vi "Pockels Cal-Cal subset info from graph.vi"(8 "error in (no error)":errorcluster, 11 "XYGraph in":refnum<vi>) -> (0 "error out":errorcluster, 1 "Cal subset info array":string[][](array[string]), 3 "XYGraph":refnum<vi>)   [LabVIEW 2020]
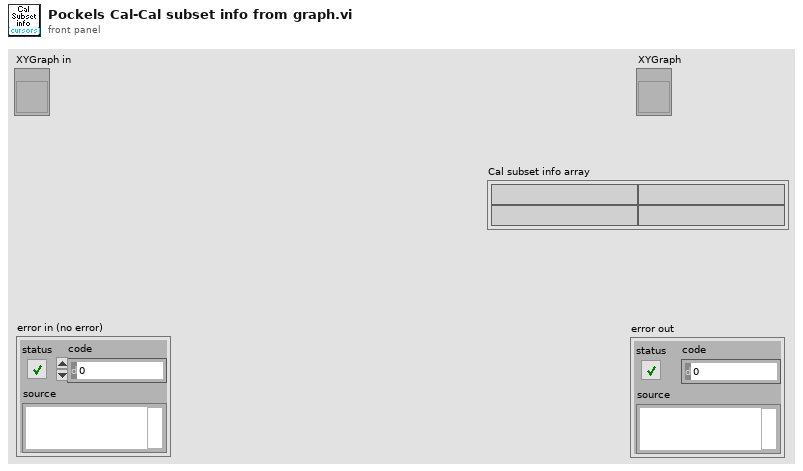
[diagram p1: front panel]
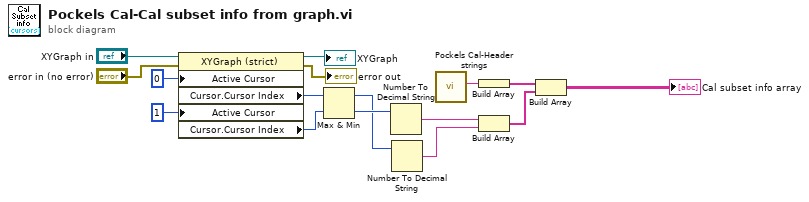
[diagram p0: block diagram]
diagram:
  n1 = property on="Property Node" class="XYGraph (strict)"(reference="XYGraph in", error in="error in (no error)", "Active Cursor"=u32 0, "Active Cursor"=u32 1) -> (reference out=→"XYGraph":refnum<vi>, error out=→"error out":errorcluster, "Cursor.Cursor Index"=w10:i32, "Cursor.Cursor Index"=w9:i32)
  n2 = Max & Min(x=w10, y=w9) -> (max(x,y)=w7:i32, min(x,y)=w8:i32)
  n3 = Number To Decimal String(number=w8) -> (decimal integer string=w15:string)  [unwired: 1 in]
  n4 = Number To Decimal String(number=w7) -> (decimal integer string=w14:string)  [unwired: 1 in]
  n5 = call "Pockels Cal-Header strings.vi"() -> ("Cal subset indexes header string"=w2:string)  [unwired: 9 in, 2 out]
  n6 = Build Array(w2) -> (w16:string[])
  n7 = Build Array(w15, w14) -> (w13:string[])
  n8 = Build Array(w16, w13) -> (→"Cal subset info array":string[][])
